vi "Callback Change Alias.vi"(6 "Variant":variant, 8 "error in (no error)":errorcluster, 9 "old values":string[][](array[string]), 10 "object ref in":T1, 11 "Table Changes":T2) -> (0 "error out":errorcluster)   [LabVIEW 2015, in "Modbus Module editor node.lvclass"]
uses:
  Modbus Module editor node.lvclass
  <vilib>/NI/DCAF/Tag Editor Core/Table API/Table Manager/Cell Change.ctl
  <vilib>/NI/DCAF/Tag Editor Core/Table API/Table Manager/object ref.ctl
  <vilib>/NI/DCAF/Tag Editor Core/Configuration Editor/Classes/Engine Parent/Engine Parent Editor Node.lvclass
  <vilib>/NI/DCAF/Tag Editor Core/Configuration Editor/Classes/Module editor node/module editor node.lvclass
  module/configuration/Modbus Module configuration.lvclass
  <vilib>/NI/Configuration Framework/serializable configuration/NISE_CEF_serializable configuration.lvclass/NISE_CEF_serializable configuration.ctl
  <vilib>/NI/Tag Bus/tag/tag descriptor.lvclass/tag descriptor.ctl
  <vilib>/Utility/LVClass/Get LV Class Name.vi
  <vilib>/NI/Configuration Framework/error generator/NISE_error generator.vi
  <vilib>/NI/Module Execution Interface/Engine Configuration/engine configuration.lvclass
  <vilib>/NI/Configuration Framework/serializable configuration/NISE_CEF_serializable configuration.lvclass
  <vilib>/NI/Tag Bus/tag/tag descriptor.lvclass
  <vilib>/NI/DCAF/Tag Editor Core/Table API/Table Manager.lvlib
  <vilib>/NI/DCAF/Tag Editor Core/Table API/Table Manager/Table Manager.lvclass
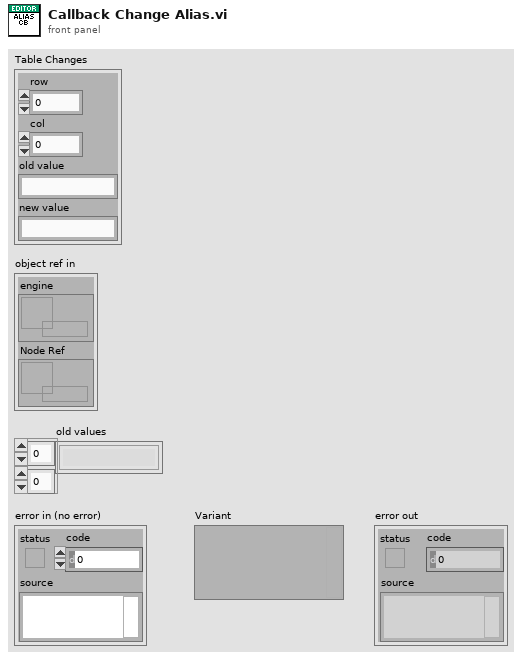
[diagram p1: front panel]
types:
  T1 = typedef "Table Manager.lvlib/Table Manager.lvclass/object ref.ctl" = cluster{"engine":refnum<data-value>, "Node Ref":refnum<data-value>}
  T2 = typedef "Table Manager.lvlib/Cell Change.ctl" = cluster{"row":i32, "col":i32, "old value":string, "new value":string}
  T3 = typedef "Modbus Module configuration.lvclass/Line.ctl" = cluster{"MB Channel":refnum<class "Modbus Module Channel.lvclass">}
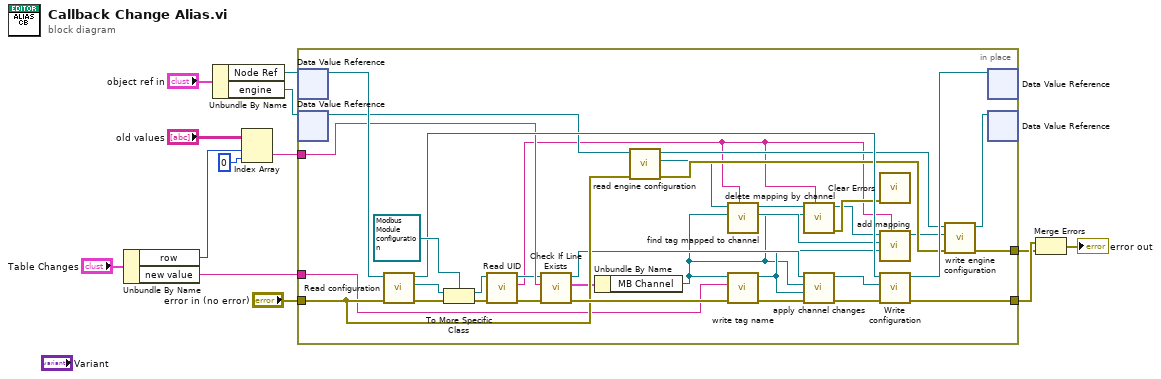
[diagram p0: block diagram]
diagram:
  n1 = Unbundle By Name("Table Changes") -> ("row"=w7:i32, "new value"=w1:string)
  n2 = Unbundle By Name("object ref in") -> ("Node Ref"=w11:refnum<data-value>, "engine"=w10:refnum<data-value>)
  n3 = Index Array(array="old values", index (row)=w7, index (col)=0 ("disabled index (col)")) -> (element=w6:string)
  n4 = in-place {
    in-place-border: w6 -> [w39]
    in-place-border: "error in (no error)" -> [w29]
    in-place-border: [w31] -> w3
    in-place-border: [w30] -> w4
    in-place-border: w1 -> [w21]
    n5 = in-place-dvr #1(w11) -> (w44:refnum<class "module editor node.lvclass">)  [unwired: 1 out]
    n6 = in-place-dvr #2(w10) -> (w40:refnum<class "Engine Parent Editor Node.lvclass">)  [unwired: 1 out]
    n7 = call-dynamic "Read configuration.vi"("error in"=w29, "NISE_CEF_serializable node in"=w44) -> ("error out"=w32:errorcluster, "configuration"=w46:refnum<class "NISE_CEF_serializable configuration.lvclass">, "NISE_CEF_serializable node out"=w43:refnum<class "module editor node.lvclass">)  [unwired: 7 in]
    n8 = To More Specific Class(target class=refnum<class "Modbus Module configuration.lvclass"> refnum ("Modbus Slave configuration in"), reference=w46, error in=w32) -> (specific class reference=w37:refnum<class "Modbus Module configuration.lvclass">, error out=w34:errorcluster)
    n9 = call <vilib>:"Read UID.vi"("error in"=w34, "configuration in"=w37) -> ("error out"=w33:errorcluster, "instance id"=w23:string, "configuration out"=w36:refnum<class "Modbus Module configuration.lvclass">)  [unwired: 7 in]
    n10 = call "Check If Line Exists.vi"("error in (no error)"=w33, "Name to locate"=w39, "Modbus Slave configuration in"=w36) -> ("error out"=w38:errorcluster, "Line out"=w15:T3, "Modbus Slave configuration out"=w20:refnum<class "Modbus Module configuration.lvclass">)  [unwired: 4 in, 2 out]
    n11 = Unbundle By Name(w15) -> ("MB Channel"=w14:refnum<class "Modbus Module Channel.lvclass">)
    n12 = call <vilib>:"read engine configuration.vi"("error in"=w29, "Engine Parent Editor Node in"=w40) -> ("error out"=w28:errorcluster, "engine configuration"=w25:refnum<class "engine configuration.lvclass">, "Engine Parent Editor Node out"=w41:refnum<class "Engine Parent Editor Node.lvclass">)  [unwired: 7 in]
    n13 = call <vilib>:"find tag mapped to channel.vi"("owner"=w23, "channel"=w14, "engine configuration in"=w25) -> ("tag"=w22:refnum<class "tag descriptor.lvclass">, "engine configuration out"=w24:refnum<class "engine configuration.lvclass">)  [unwired: 6 in, 1 out]
    n14 = call <vilib>:"write tag name.vi"("error in"=w38, "name"=w21, "system tag in"=w14) -> ("error out"=w17:errorcluster, "system tag out"=w18:refnum<class "Modbus Module Channel.lvclass">)  [unwired: 7 in]
    n15 = call <vilib>:"delete mapping by channel.vi"("owner ID"=w23, "channel"=w14, "engine configuration in"=w24) -> ("error out"=w35:errorcluster, "engine configuration out"=w27:refnum<class "engine configuration.lvclass">)  [unwired: 7 in]
    n16 = call "apply channel changes.vi"("error in"=w17, "new channel"=w18, "old channel"=w14, "Modbus Slave configuration in"=w20) -> ("error out"=w16:errorcluster, "Modbus Slave configuration out"=w19:refnum<class "Modbus Module configuration.lvclass">)  [unwired: 6 in]
    n17 = call <vilib>:"Clear Errors.vi"("error in (no error)"=w35) -> ()  [unwired: 5 in, 2 out]
    n18 = call-dynamic "add mapping.vi"("owner ID"=w23, "channel"=w18, "tag descriptor"=w22, "engine configuration"=w27) -> ("engine configuration out"=w26:refnum<class "engine configuration.lvclass">)  [unwired: 6 in, 1 out]
    n19 = call-dynamic "Write configuration.vi"("error in"=w16, "configuration"=w19, "NISE_CEF_serializable node in"=w43) -> ("error out"=w30:errorcluster, "NISE_CEF_serializable node out"=w45:refnum<class "module editor node.lvclass">)  [unwired: 7 in]
    n20 = call <vilib>:"write engine configuration.vi"("error in"=w28, "engine configuration"=w26, "Engine Parent Editor Node in"=w41) -> ("error out"=w31:errorcluster, "Engine Parent Editor Node out"=w42:refnum<class "Engine Parent Editor Node.lvclass">)  [unwired: 7 in]
    n21 = in-place-dvr #1(w45) -> ()  [unwired: 2 out]
    n22 = in-place-dvr #2(w42) -> ()  [unwired: 2 out]
  }
  n23 = Merge Errors(w4, w3) -> (→"error out":errorcluster)
